vi "Connected to a Star.vi"(10 "Digit Array":T1[](array[typedef]), 11 "Unsigned Byte Array":u8[][](array[numeric])) -> (2 "Connected Star Array":T1[](array[typedef]), 3 "Connected to Star":bool)   [LabVIEW 2023]
uses:
  Cluster Digit.ctl
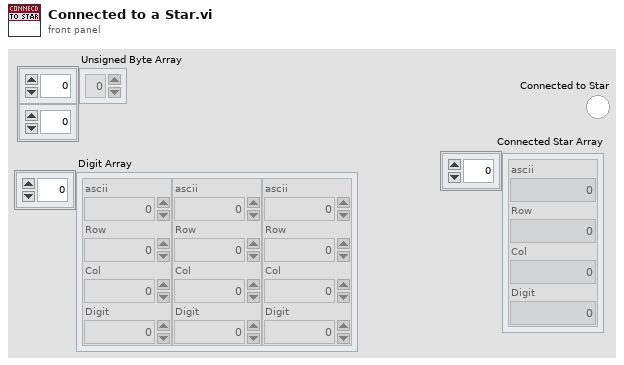
[diagram p1: front panel]
types:
  T1 = typedef "Cluster Digit.ctl" = cluster{"ascii":u8, "Row":i32, "Col":i32, "Digit":i32}
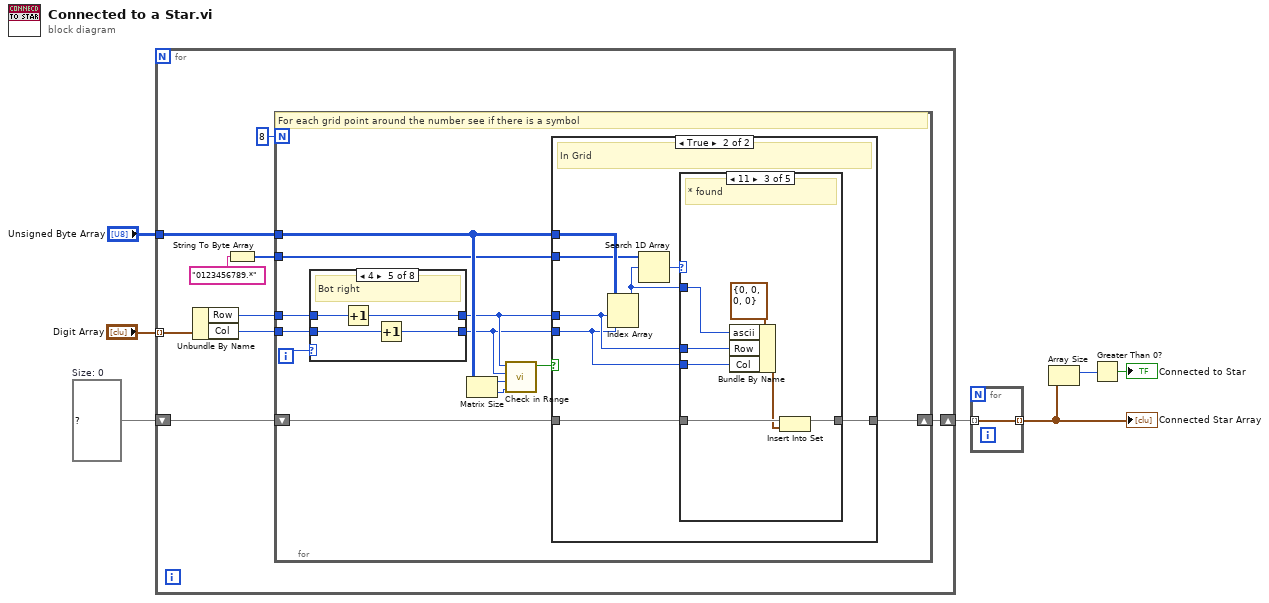
[diagram p0: block diagram]
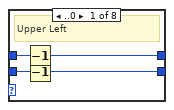
[diagram p2: hidden frame]
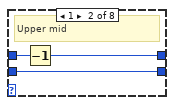
[diagram p3: hidden frame]
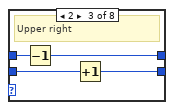
[diagram p4: hidden frame]
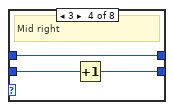
[diagram p5: hidden frame]
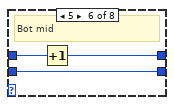
[diagram p6: hidden frame]
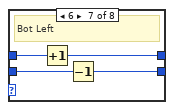
[diagram p7: hidden frame]
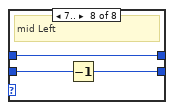
[diagram p8: hidden frame]
diagram:
  w3 = set{T1} {}  # Size: 0
  n1 = for {
    tunnel: "Digit Array" -> [w16] mode=indexing
    tunnel: "Unsigned Byte Array" -> [w14]
    shift-right: [w8] -> w2
    shift-left: w3 -> [w9]
    n2 = Unbundle By Name(w16) -> ("Row"=w13:i32, "Col"=w12:i32)
    n3 = String To Byte Array(string="0123456789.*" ("String")) -> (unsigned byte array=w11:u8[])
    n4 = for {
      N: 8 -> [_]
      tunnel: w11 -> [w19]
      tunnel: w14 -> [w26]
      tunnel: w13 -> [w28]
      tunnel: w12 -> [w27]
      shift-right: [w17] -> w8
      shift-left: w9 -> [w18]
      i -> [w20]
      # "For each grid point around the number see if there is a symbol"
      n5 = case shown="4" w20 {
        tunnel: w28 -> [w32 w35 w39 w40 w44 w49 w53 w54]
        tunnel: w27 -> [w31 w33 w37 w42 w46 w47 w51 w56]
        tunnel: [w30 w34 w38 w40 w43 w48 w52 w54] -> w24
        tunnel: [w29 w33 w36 w41 w45 w47 w50 w55] -> w22
        frame ..0 {
          # "Upper Left"
          n6 = Decrement(x=w32) -> (x-1=w30:i32)
          n7 = Decrement(x=w31) -> (x-1=w29:i32)
        }
        frame 1 {
          # "Upper mid"
          n8 = Decrement(x=w35) -> (x-1=w34:i32)
        }
        frame 2 {
          # "Upper right"
          n9 = Decrement(x=w39) -> (x-1=w38:i32)
          n10 = Increment(x=w37) -> (x+1=w36:i32)
        }
        frame 3 {
          # "Mid right"
          n11 = Increment(x=w42) -> (x+1=w41:i32)
        }
        frame 4 {
          # "Bot right"
          n12 = Increment(x=w44) -> (x+1=w43:i32)
          n13 = Increment(x=w46) -> (x+1=w45:i32)
        }
        frame 5 {
          # "Bot mid"
          n14 = Increment(x=w49) -> (x+1=w48:i32)
        }
        frame 6 {
          # "Bot Left"
          n15 = Increment(x=w53) -> (x+1=w52:i32)
          n16 = Decrement(x=w51) -> (x-1=w50:i32)
        }
        frame 7.. {
          # "mid Left"
          n17 = Decrement(x=w56) -> (x-1=w55:i32)
        }
      }
      n18 = Matrix Size(0:w26) -> (1:w23:i32, 2:w21:i32)
      n19 = call "Check in Range.vi"("number of col"=w21, "number of rows"=w23, "col"=w22, "row"=w24) -> ("in range"=w25:bool)  [unwired: 7 in]
      n20 = case shown="True" w25 {
        tunnel: w26 -> [_ w65]
        tunnel: w22 -> [_ w60]
        tunnel: w24 -> [_ w61]
        tunnel: w19 -> [_ w64]
        tunnel: w18 -> [w57 w59]
        tunnel: [w57 w58] -> w17
        frame False {
          # "Out of Grid"
        }
        frame True {
          # "In Grid"
          n21 = Index Array(array=w65, index (row)=w61, index (col)=w60) -> (element=w62:u8)
          n22 = Search 1D Array(1D array=w64, element=w62) -> (index of element=w63:i32)  [unwired: 1 in]
          n23 = case shown="11" w63 {
            tunnel: w62 -> [_ _ w73 _ _]
            tunnel: w61 -> [_ _ w72 _ _]
            tunnel: w60 -> [_ _ w71 _ _]
            tunnel: w59 -> [w66 w67 w70 w75 w76]
            tunnel: [w66 w67 w69 w75 w76] -> w58
            frame 0..9 {
              # "Number Found"
            }
            frame 10 {
              # ". found"
            }
            frame 11 {
              # "* found"
              n24 = Bundle By Name(cluster=T1 {"ascii"=0, "Row"=0, "Col"=0, "Digit"=0} ("Digit"), "ascii"=w73, "Row"=w72, "Col"=w71) -> (w68:T1)
              n25 = Insert Into Set(10:w68, 11:w70) -> (3:w69:set{T1})  [unwired: 1 out]
            }
            frame 12.. {
              # "nothing"
            }
            frame ..-1 {
              # "symbol found"
            }
          }
        }
      }
    }
  }
  n26 = for {
    tunnel: w2 -> [w77] mode=indexing
    tunnel: [w77] -> w1 mode=indexing
  }
  "Connected Star Array" <- w1
  n27 = Array Size(array=w1) -> (size(s)=w5:i32)
  n28 = Greater Than 0?(x=w5) -> (x > 0?=→"Connected to Star":bool)
